vi "Stop.vi"(7 "LabVIEW Web Service Request":refnum<class "Web Request.lvclass">) -> ()   [LabVIEW 2023]
uses:
  <vilib>/wsapi/Web Request.lvclass
panel:
  # "Use the Web Service Request input terminal to call the VIs on the Web Services palette. Do not remove it from the connector pane unless you don't need access to the palette."
  # "Each additional control wired to the connector pane will be available as an input in the URL. To include an indicator in terminal-mode output (the default setting), it must also be wired to the connector pane."
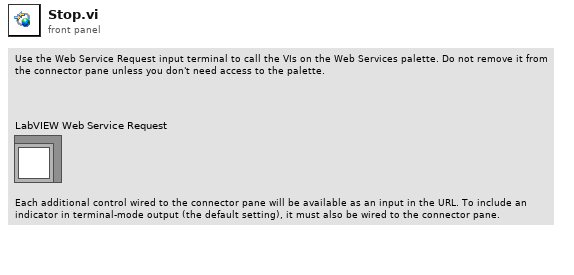
[diagram p1: front panel]
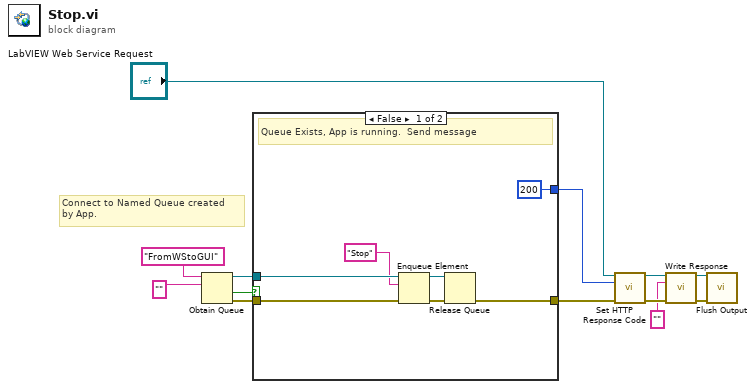
[diagram p0: block diagram]
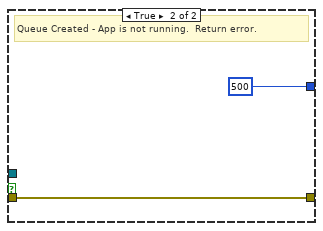
[diagram p2: hidden frame]
diagram:
  # "Connect to Named Queue created\nby App."
  n1 = Obtain Queue(name (unnamed)="FromWStoGUI", element data type="") -> (queue out=w10:refnum<queue>, created new?=w11:bool, error out=w9:errorcluster)  [unwired: 3 in]
  n2 = case shown="False" w11 {
    tunnel: w10 -> [w20 _]
    tunnel: w9 -> [w19 w22]
    tunnel: [w15 w22] -> w7
    tunnel: [200 500] -> w6
    frame False {
      # "Queue Exists, App is running.  Send message"
      n3 = Enqueue Element(queue=w20, element="Stop", error in (no error)=w19) -> (queue out=w17:refnum<queue>, error out=w16:errorcluster)  [unwired: 1 in, 1 out]
      n4 = Release Queue(queue=w17, error in (no error)=w16) -> (error out=w15:errorcluster)  [unwired: 1 in, 2 out]
    }
    frame True {
      # "Queue Created - App is not running.  Return error."
    }
  }
  n5 = call <vilib>:"Set HTTP Response Code.vi"("LabVIEW Web Service Request"="LabVIEW Web Service Request", "response code (200)"=w6, "error in (no error)"=w7) -> ("LabVIEW Web Service Request out"=w5:refnum<class "Web Request.lvclass">, "error out"=w4:errorcluster)  [unwired: 11 in]
  n6 = call <vilib>:"Write Response.vi"("LabVIEW Web Service Request"=w5, "response string"="", "error in (no error)"=w4) -> ("LabVIEW Web Service Request out"=w2:refnum<class "Web Request.lvclass">, "error out"=w1:errorcluster)  [unwired: 11 in]
  n7 = call <vilib>:"Flush Output.vi"("LabVIEW Web Service Request"=w2, "error in (no error)"=w1) -> ()  [unwired: 12 in, 2 out]
